vi "getMacAddress.vi"(8 "error in":errorcluster, 10 "Mac Adress in":string, 11 "connection ID":refnum<k5>) -> (0 "error out":errorcluster, 2 "Mac Adress out":string, 3 "connection ID":refnum<k5>)   [LabVIEW 2016]
panel:
  in  "Get Command":string="com.attocube.system.getMacAddress"
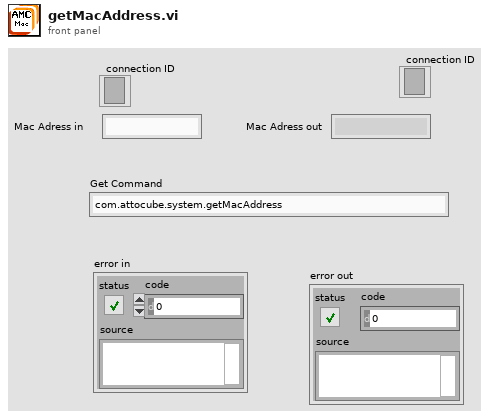
[diagram p1: front panel]
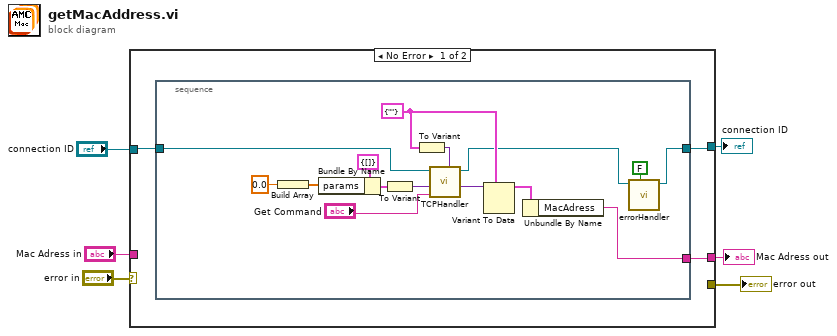
[diagram p0: block diagram]
diagram:
  n1 = case shown="No Error" "error in" {
    selector: "error in" -> [_ w27]
    tunnel: [_ w27] -> w1
    tunnel: "Mac Adress in" -> [_ w26]
    tunnel: [w8 w26] -> w5
    tunnel: [w9 w25] -> w4
    tunnel: "connection ID" -> [w7 w25]
    frame No Error {
      n2 = stacked-sequence {
        tunnel: [w10] -> w9
        tunnel: w7 -> [w17]
        tunnel: [w14] -> w8
        frame #0 {
          w15 = cluster{"MacAdress":string} {"MacAdress"=""} ("input cluster")
          n3 = Build Array(0.0 ("element")) -> (w21:dbl[])
          n4 = Bundle By Name(cluster=cluster{"params":i16[]} {"params"=[]} ("input cluster"), "params"=w21) -> (w22:cluster{"params":i16[]})
          n5 = To Variant(anything=w22) -> (Variant=w23:variant)
          n6 = To Variant(anything=w15) -> (Variant=w16:variant)
          n7 = call "TCPHandler.vi"("result Types"=w16, "method"="Get Command", "params"=w23, "connection ID"=w17) -> ("result"=w19:variant, "connection ID"=w11:refnum<k5>)  [unwired: 5 in, 1 out]
          n8 = Variant To Data(type=w15, Variant=w19) -> (data=w24:cluster{"MacAdress":string})  [unwired: 1 in, 1 out]
          n9 = Unbundle By Name(w24) -> ("MacAdress"=w14:string)
          n10 = call "errorHandler.vi"("show popup"=FALSE, "connection ID"=w11) -> ("connection ID"=w10:refnum<k5>)  [unwired: 8 in, 1 out]
        }
      }
    }
    frame Error {
    }
  }
  "error out" <- w1
  "Mac Adress out" <- w5
  "connection ID" <- w4
